vi "add_pdf_extension_unique.vi"(11 "PDF File Name in":string) -> (3 "PDF File Name out":string)   [LabVIEW 2020, in "Linearisierung v2.lvlib" / "Protokoll.lvlib"]
uses:
  Protokoll.lvlib
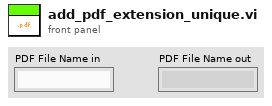
[diagram p1: front panel]
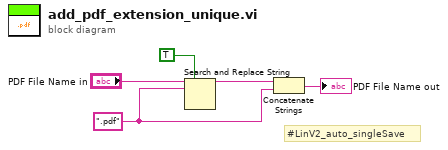
[diagram p0: block diagram]
diagram:
  w2 = ".pdf"
  # "#LinV2_auto_singleSave"
  n1 = Search and Replace String(replace all?=TRUE ("Alle ersetzen? (F)"), input string="PDF File Name in", search string=w2) -> (result string=w3:string)  [unwired: 5 in, 3 out]
  n2 = Concatenate Strings(w3, w2) -> (→"PDF File Name out":string)
